vi "3.1.vi"() -> ()   [LabVIEW 2015]
panel:
  out "平方的和":dbl
  in  "数组":dbl[](array[numeric])
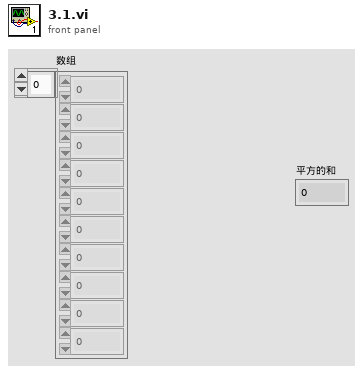
[diagram p1: front panel]
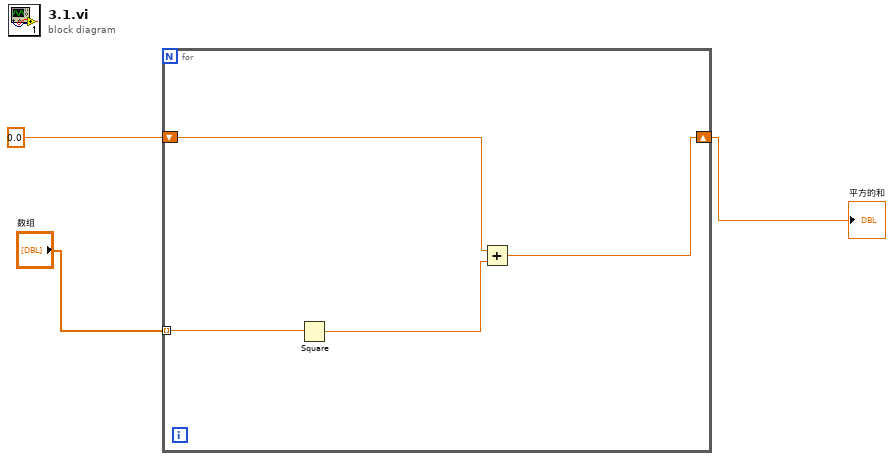
[diagram p0: block diagram]
diagram:
  n1 = for {
    tunnel: "数组" -> [w6] mode=indexing
    shift-right: [w4] -> w1
    shift-left: 0.0 -> [w5]
    n2 = Square(x=w6) -> (x^2=w7:dbl)
    n3 = Add(x=w5, y=w7) -> (x+y=w4:dbl)
  }
  "平方的和" <- w1
